vi "Ordered Query.vi"(8 "error in (no error)":errorcluster, 9 "Parameters":map{string, variant}(c390), 10 "Query":string, 11 "Sqlite Database Manager in":refnum<class "Sqlite Database Manager.lvclass">) -> (0 "error out":errorcluster, 1 "Rows":cluster{"Column":string, "Value":variant}[][](array[cluster]), 3 "Sqlite Database Manager out":refnum<class "Sqlite Database Manager.lvclass">)   [LabVIEW 2019, in "HierDAL Library.lvlib" / "Database.lvlib" / "Sqlite Database Manager.lvclass"]
doc: "Executes a SQL query and retrieves the results preserving the column order.\nParameters are used to safely inject values into the SQL command, preventing SQL injection attacks.\nIt ensure that inputs are only ever treated as literal values and never executed.\n\nParameters can be prefixed with either :, @, or $.\ne.g.\n\"\"\"\n SELECT country, year \n FROM generals\n WHERE name = @name\n\"\"\"\n\n<b>Query</b> - The SQL query to execute.\n<b>Parameters</b> - A map of parameter (must have prefix) names and their corresponding values.\n<b>Rows</b> - A 2d array of key-values, with each row representing a row of column-value pairs."
uses:
  Sqlite Database Manager.lvclass
  Sqlite Database Manager.lvclass/Sqlite Database Manager.ctl
  System.Data.SQLite
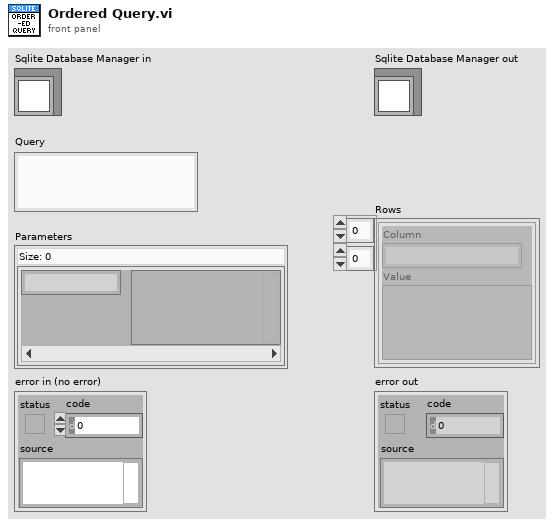
[diagram p1: front panel]
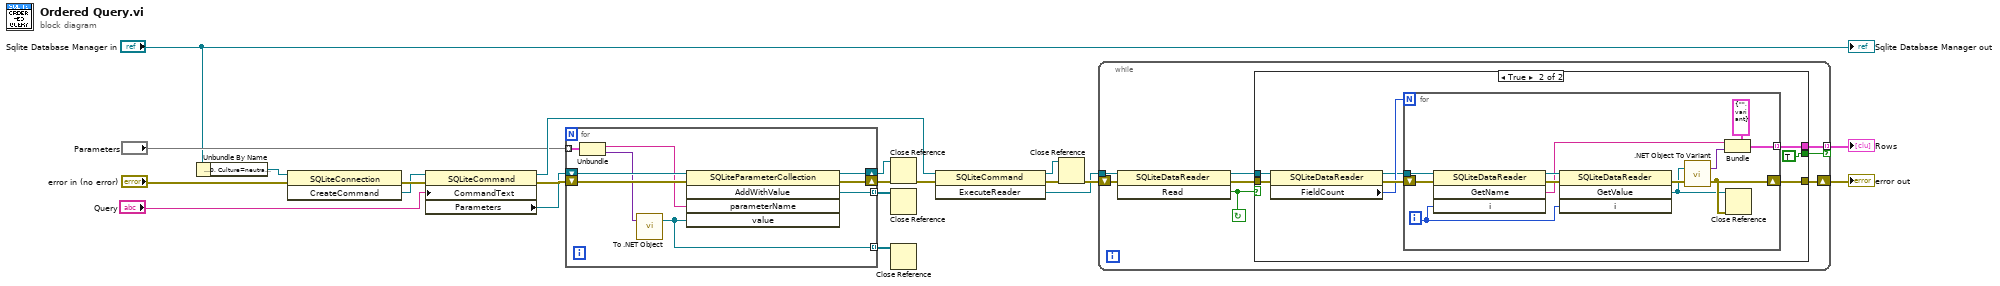
[diagram p0: block diagram]
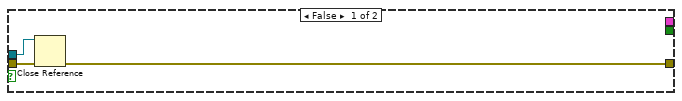
[diagram p2: hidden frame]
diagram:
  n1 = Unbundle By Name("Sqlite Database Manager in") -> ("Connection"=w21:refnum<k24>)
  n2 = invoke class="SQLiteConnection" method="CreateCommand"(reference=w21, error in="error in (no error)") -> (error out=w20:errorcluster, "CreateCommand"=w19:refnum<k24>)  [unwired: 1 in, 1 out]
  n3 = property class="SQLiteCommand"(reference=w19, error in=w20, "CommandText"="Query") -> (reference out=w11:refnum<k24>, error out=w18:errorcluster, "Parameters"=w17:refnum<k24>)
  n4 = for {
    shift-right: [w26] -> w13
    shift-left: w17 -> [w28]
    tunnel: "Parameters" -> [w29] mode=indexing
    shift-right: [w27] -> w16
    shift-left: w18 -> [w30]
    tunnel: [w25] -> w14 mode=indexing
    tunnel: [w24] -> w15 mode=indexing
    n5 = Unbundle(w29) -> ("Parameter"=w22:string, "Value"=w23:variant)
    n6 = call <vilib>:"To .NET Object.vi"("anything"=w23) -> (".NET object"=w24:refnum<k24>)  [unwired: 1 in, 1 out]
    n7 = invoke class="SQLiteParameterCollection" method="AddWithValue"(reference=w28, error in=w30, "parameterName"=w22, "value"=w24) -> (reference out=w26:refnum<k24>, error out=w27:errorcluster, "AddWithValue"=w25:refnum<k24>)  [unwired: 1 in, 2 out]
  }
  n8 = Close Reference(reference=w13, error in (no error)=w16) -> (error out=w12:errorcluster)
  n9 = Close Reference(reference=w14) -> ()  [unwired: 1 in, 1 out]
  n10 = Close Reference(reference=w15) -> ()  [unwired: 1 in, 1 out]
  n11 = invoke class="SQLiteCommand" method="ExecuteReader"(reference=w11, error in=w12) -> (reference out=w9:refnum<k24>, error out=w10:errorcluster, "ExecuteReader"=w4:refnum<k24>)  [unwired: 1 in]
  n12 = Close Reference(reference=w9, error in (no error)=w10) -> (error out=w5:errorcluster)
  n13 = while {
    shift-right: [w33] -> w1
    shift-left: w5 -> [w38]
    tunnel: w4 -> [w37]
    tunnel: [w32] -> w2 mode=indexing if=w31
    stop <- w36 continue-if-true
    n14 = invoke class="SQLiteDataReader" method="Read"(reference=w37, error in=w38) -> (reference out=w34:refnum<k24>, error out=w35:errorcluster, "Read"=w36:bool)  [unwired: 1 in]
    n15 = case shown="True" w36 {
      tunnel: w35 -> [w41 w49]
      tunnel: w34 -> [w40 w48]
      tunnel: [w39 w45] -> w33
      tunnel: [_ w42] -> w32
      tunnel: [_ TRUE] -> w31
      frame False {
        n16 = Close Reference(reference=w40, error in (no error)=w41) -> (error out=w39:errorcluster)
      }
      frame True {
        n17 = property class="SQLiteDataReader"(reference=w48, error in=w49) -> (reference out=w44:refnum<k24>, error out=w47:errorcluster, "FieldCount"=w46:i32)
        n18 = for {
          N: w46 -> [_]
          shift-right: [w56] -> w45
          shift-left: w47 -> [w61]
          tunnel: w44 -> [w60]
          tunnel: [w50] -> w42 mode=indexing
          i -> [w58]
          n19 = invoke class="SQLiteDataReader" method="GetName"(reference=w60, error in=w61, "i"=w58) -> (reference out=w54:refnum<k24>, error out=w59:errorcluster, "GetName"=w52:string)  [unwired: 1 in, 1 out]
          n20 = invoke class="SQLiteDataReader" method="GetValue"(reference=w54, error in=w59, "i"=w58) -> (error out=w57:errorcluster, "GetValue"=w55:refnum<k24>)  [unwired: 1 in, 2 out]
          n21 = call <vilib>:".NET Object To Variant.vi"("error in (no error)"=w57, ".NET object"=w55) -> ("error out"=w56:errorcluster, "variant"=w51:variant)
          n22 = Bundle(cluster=cluster{"Column":string, "Value":variant} {"Column"="", "Value"=variant}, "Column"=w52, "Value"=w51) -> (w50:cluster{"Column":string, "Value":variant})
          n23 = Close Reference(reference=w55, error in (no error)=w56) -> ()  [unwired: 1 out]
        }
      }
    }
  }
  "error out" <- w1
  "Rows" <- w2
  "Sqlite Database Manager out" <- "Sqlite Database Manager in"
